vi "Slam.vi"() -> ()   [LabVIEW 2017]
uses:
  Control Globals.vi
  gyro/Gyro Globals.vi
  <vilib>/Platform/TimedLoop/XDataNode/wakeup.ctl
  <vilib>/Platform/TimedLoop/XDataNode/XDNodeRunTimeDep.lvlib
  <vilib>/Platform/TimedLoop/XDataNode/nitl_modes.ctl
  <vilib>/Platform/TimedLoop/XDataNode/timing_clust.ctl
  <vilib>/Platform/TimedLoop/XDataNode/XDataNode.xnode
  <vilib>/robotics/Steering/Steering Frame/NI_Robotics_Steering Frame.lvclass
  <vilib>/robotics/Steering/Steering Frame/Apply Steering Frame Velocity to Motors.vi
panel:
  out "Estimated Pose (Degrees)":cluster{"X":dbl, "Y":dbl, "R":dbl}
  in  "Desired Velocity":dbl[](array[numeric])=[0.0, 0.0, 0.0]
  out "Gyro Bias":cluster{"X":dbl, "Y":dbl, "Z":dbl}={"X"=0.039458598891488325, "Y"=-0.012762257416847495, "Z"=-0.06349169800034307}
  out "Slam Run Time":u32
  out "Intensity Graph":u16[][](graph)
  in  "stop":bool
  out "XY Graph":cluster{"X":dbl[], "Y":dbl[]}[](graph)
  out "Lidar Run Time":u32
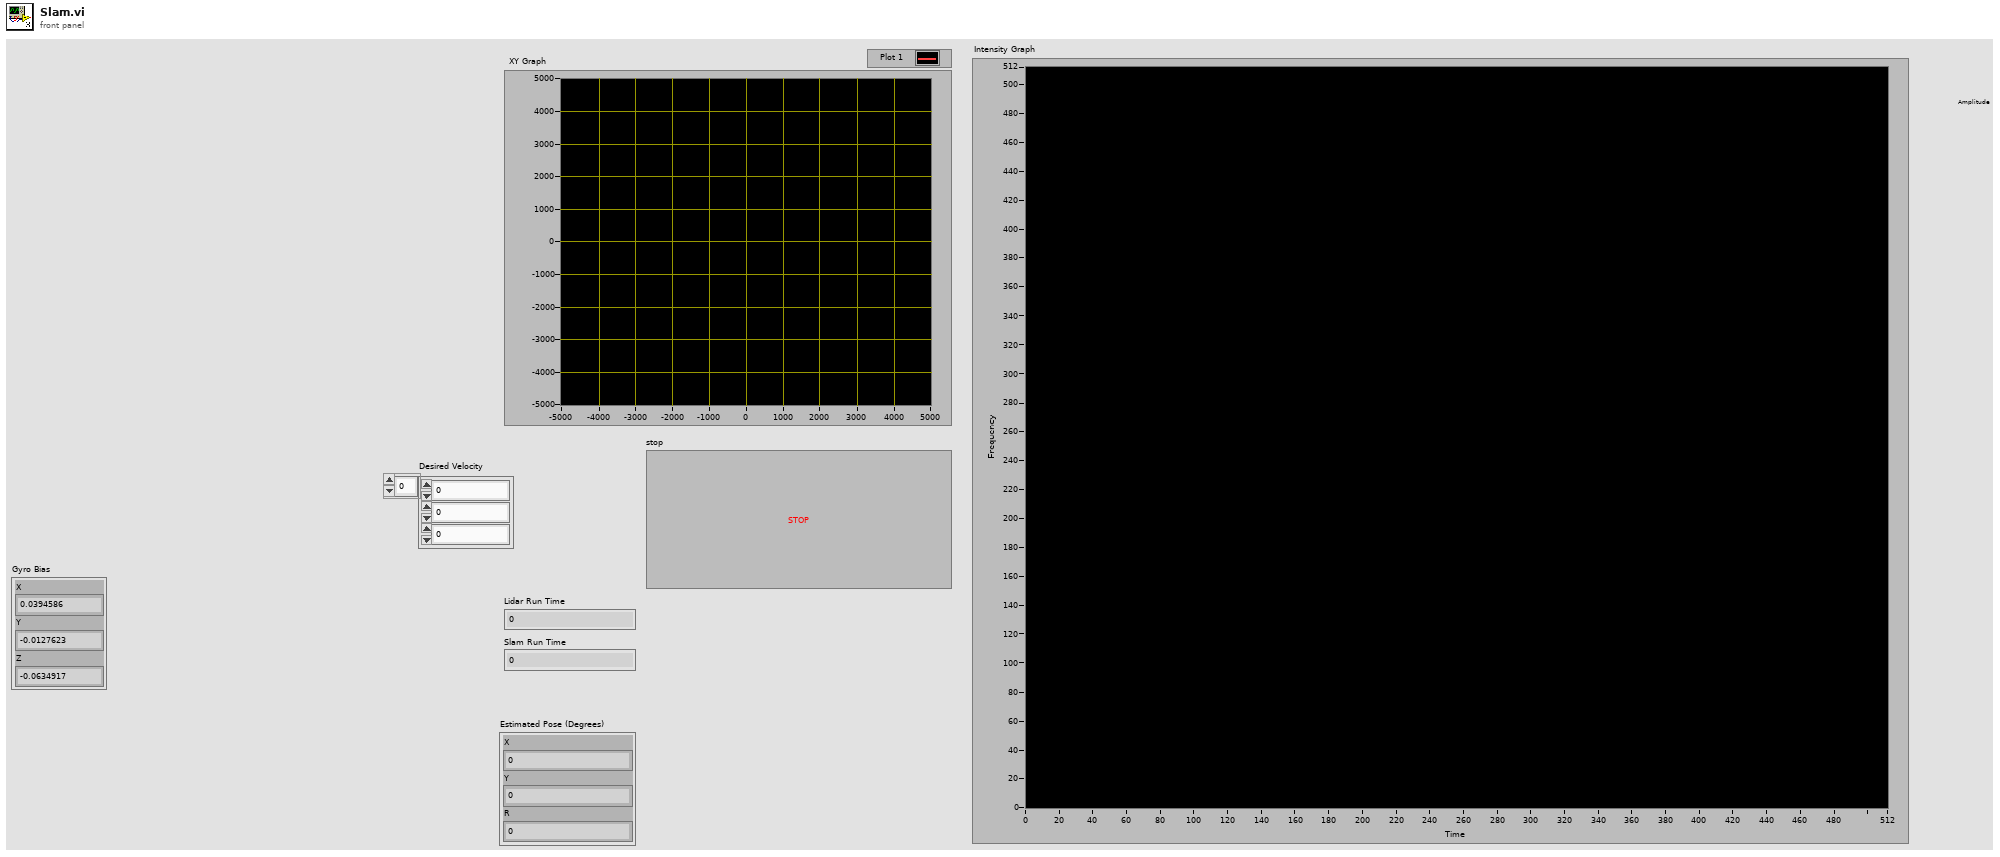
[diagram p1: front panel]
types:
  T1 = cluster{dbl[], dbl[], "Estimated Pose Delta":cluster{"X":dbl, "Y":dbl, "R":dbl}}
  T2 = typedef "XDNodeRunTimeDep.lvlib/timing_clust.ctl" = cluster{"Expected End [f-1]":u64, "Actual End [f-1]":u64, "Finished Late? [f-1]":bool, "Expected End [i-1]":u64, "Actual End [i-1]":u64, "Finished Late? [i-1]":bool, "Expected Start [i]":u64, "Actual Start [i]":u64, "Expected Start [f]":u64, "Actual Start [f]":u64, "Source Name":string, "Structure Name":string, "Period":i64, "Deadline":i64, "Offset":i64, "Start":i64, "Priority":i32, "Timeout":i32, "Mode":T3, "Wakeup Reason":T4, "Error":errorcluster, "Source Type":string, "Secondary Source Type":string, "Global End Time":u64, "Global Start Time":u64, "Frame Duration":u64, "Iteration Duration":u64, "Assigned CPU":i32, "I/O Scan Engine Mode":u32}
  T3 = typedef "XDNodeRunTimeDep.lvlib/nitl_modes.ctl" = enum32{"No Change", "Process missed periods, maintain original phase", "Discard missed periods, maintain original phase", "Process missed periods, ignore original phase", "Discard missed periods, ignore original phase"}
  T4 = typedef "XDNodeRunTimeDep.lvlib/wakeup.ctl" = enum32{"Normal", "Aborted", "Asynchronous wakeup", "Timing source error", "Timed loop error", "Timeout"}
  T5 = typedef "I2C.lvlib/I2C Reference.ctl" = cluster{"myRIO Reference":T6, "I2C Channels Enum":T10, "I2C Configuration":T11}
  T6 = typedef "myRIO Generic Hardware Reference.ctl" = cluster{"myRIO Model":T7, "myRIO Hardware Reference":T8}
  T7 = typedef "Hardware Version Enum.ctl" = enum16{"Unknown", "myRIO-1900", "myRIO-1950", "roboRIO", "NI ELVIS RIO CM"}
  T8 = typedef "myRIO v1.0 Reference.ctl" = cluster{"Generic FPGA Reference":T9, "Allow multiple opens":bool}
  T9 = typedef "Generic FPGA Reference.ctl" = refnum<k20>
  T10 = typedef "I2C Channels Enum.ctl" = enum16{"Not Connected", "A/I2C", "B/I2C", "I2C/I2C"}
  T11 = typedef "I2C.lvlib/I2C Configuration.ctl" = cluster{"I2C Transfer Rate":T12}
  T12 = typedef "I2C.lvlib/I2C Transfer Rate.ctl" = enum16{"Standard mode (100 kbps)", "Fast mode (400 kbps)"}
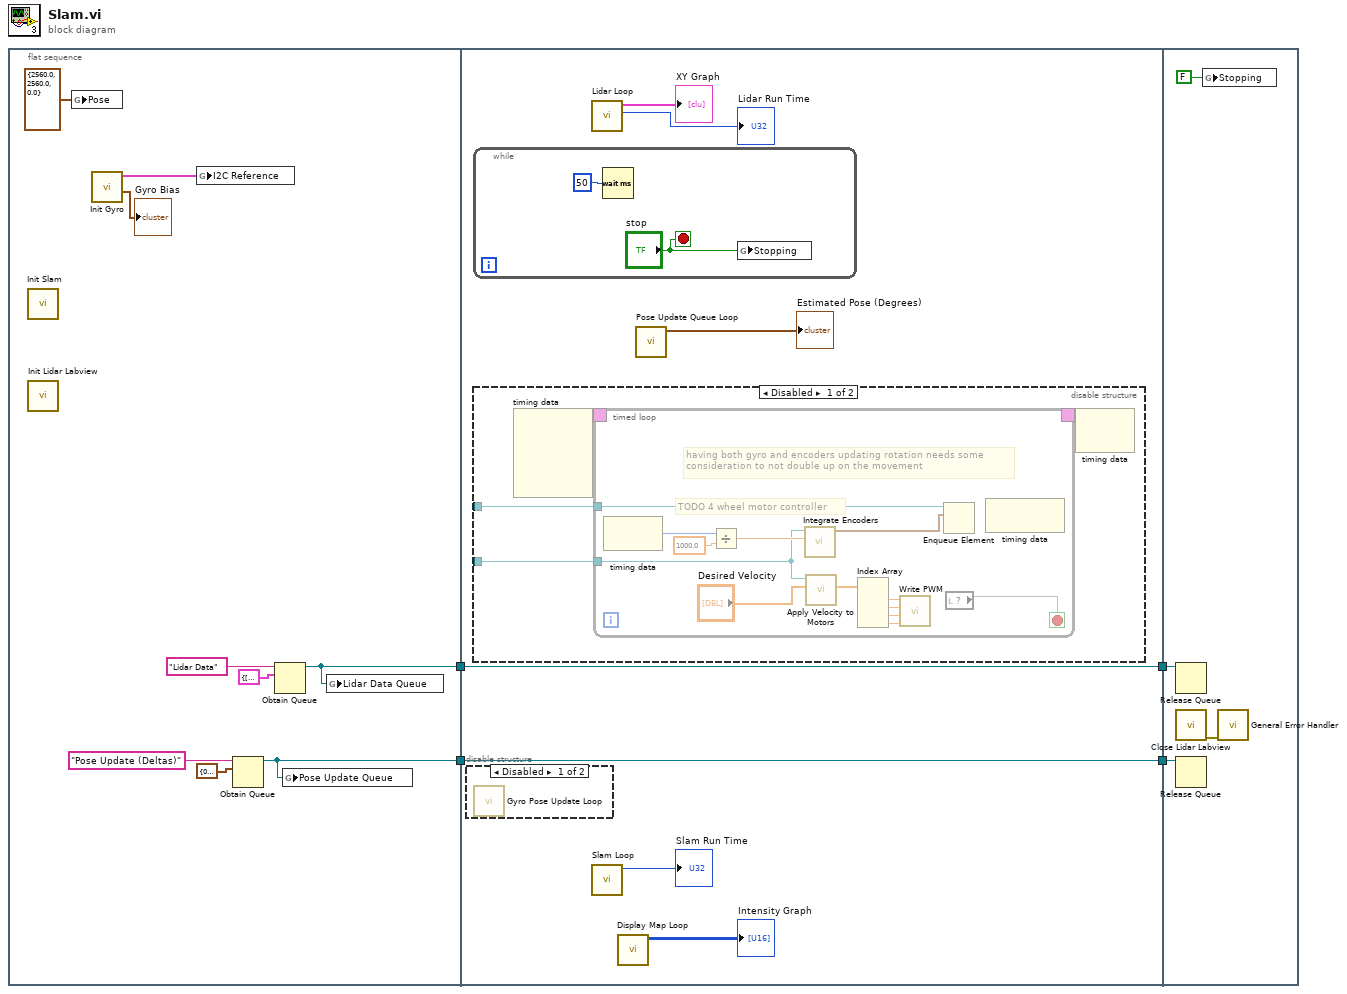
[diagram p0: block diagram]
diagram:
  n1 = flat-sequence {
    tunnel: [w8] -> w4
    tunnel: [w7] -> w3
    tunnel: w4 -> [w20]
    tunnel: w3 -> [w19]
    tunnel: [w20] -> w2
    tunnel: [w19] -> w1
    tunnel: w2 -> [w47]
    tunnel: w1 -> [w46]
    frame #0 {
      n2 = call "Init Slam.vi"() -> ()  [unwired: 12 in]
      n3 = call "Init Lidar Labview.vi"() -> ()  [unwired: 11 in, 1 out]
      n4 = global write "Control Globals.vi" "Pose"(cluster{"X":dbl, "Y":dbl, "R":dbl} {"X"=2560.0, "Y"=2560.0, "R"=0.0} ("Estimated Pose")) -> ()
      n5 = call "Init Gyro.vi"() -> ("Gyro Bias"=→"Gyro Bias":cluster{"X":dbl, "Y":dbl, "Z":dbl}, "I2C Ref Out"=w6:T5)  [unwired: 9 in, 1 out]
      n6 = global write "Gyro Globals.vi" "I2C Reference"(w6) -> ()
      n7 = Obtain Queue(name (unnamed)="Pose Update (Deltas)", element data type=cluster{"X":dbl, "Y":dbl, "R":dbl} {"X"=0.0, "Y"=0.0, "R"=0.0} ("Estimated Pose Delta")) -> (queue out=w7:refnum<queue>)  [unwired: 3 in, 2 out]
      n8 = Obtain Queue(name (unnamed)="Lidar Data", element data type=T1 {[], [], "Estimated Pose Delta"={"X"=0.0, "Y"=0.0, "R"=0.0}} ("output cluster")) -> (queue out=w8:refnum<queue>)  [unwired: 3 in, 2 out]
      n9 = global write "Control Globals.vi" "Pose Update Queue"(w7) -> ()
      n10 = global write "Control Globals.vi" "Lidar Data Queue"(w8) -> ()
    }
    frame #1 {
      n11 = disable-structure shown="Disabled" {
        frame Disabled {
          n12 = call "Gyro Pose Update Loop.vi"() -> ()  [unwired: 12 in]
        }
        frame Enabled {
        }
      }
      n13 = while {
        stop <- "stop" stop-if-true
        n14 = Wait (ms)(milliseconds to wait=u32 50) -> ()  [unwired: 1 out]
        n15 = global write "Control Globals.vi" "Stopping"("stop") -> ()
      }
      n16 = disable-structure shown="Disabled" {
        disable-tunnel: _ -> [w24 _]
        disable-tunnel: _ -> [w23 _]
        frame Disabled {
          n17 = node-c288() -> (w26:T2)  [unwired: 4 in]
          n18 = timed-loop {
            timing: w26 -> [_]
            timing-out: [_] -> w25
            tunnel: w24 -> [w32]
            tunnel: w23 -> [w28]
            stop <- w39 stop-if-true
            # "having both gyro and encoders updating rotation needs some\nconsideration to not double up on the movement"
            # "TODO 4 wheel motor controller"
            n19 = node-c288() -> (w36:i64)  [unwired: 1 in]
            n20 = Divide(x=w36, y=1000.0) -> (x/y=w37:dbl)
            n21 = call "Integrate Encoders.vi"("dt"=w37, "NI_Robotics_Steering Frame in"=w32) -> ("Estimated Pose Delta"=w27:cluster{dbl, dbl, dbl})  [unwired: 9 in]
            n22 = call-poly <vilib>:"Apply Velocity to Motors.vi"("steering frame velocity"="Desired Velocity", "steering frame in"=w32) -> ("ccw motor velocity setpoints"=w34:dbl[])  [unwired: 5 in, 4 out]
            n23 = Index Array(array=w34) -> (element #1=w35:dbl, element #2=w31:dbl, element #3=w30:dbl, element #4=w29:dbl)  [unwired: 4 in]
            n24 = call "Write PWM.vi"("Back Right"=w29, "Front Right"=w30, "Back Left"=w31, "Front Left"=w35) -> ()  [unwired: 8 in]
            n25 = Enqueue Element(queue=w28, element=w27) -> ()  [unwired: 2 in, 3 out]
            n26 = local read item#-1() -> (w39)
            n27 = node-c288() -> ()  [unwired: 1 in, 1 out]
          }
          n28 = node-c288(w25) -> ()  [unwired: 1 out]
        }
        frame Enabled {
        }
      }
      n29 = call "Lidar Loop.vi"() -> ("Lidar Run Time"=→"Lidar Run Time":u32, "XY Graph"=→"XY Graph":cluster{"X":dbl[], "Y":dbl[]}[])  [unwired: 10 in]
      n30 = call "Slam Loop.vi"() -> ("slam run time"=→"Slam Run Time":u32)  [unwired: 11 in]
      n31 = call "Display Map Loop.vi"() -> ("Intensity Graph"=→"Intensity Graph":u16[][])  [unwired: 11 in]
      n32 = call "Pose Update Queue Loop.vi"() -> ("Estimated Pose (Degrees)"=→"Estimated Pose (Degrees)":cluster{"X":dbl, "Y":dbl, "R":dbl})  [unwired: 11 in]
    }
    frame #2 {
      n33 = Release Queue(queue=w47) -> ()  [unwired: 2 in, 3 out]
      n34 = call "Close Lidar Labview.vi"() -> ("error out"=w48:errorcluster)  [unwired: 11 in]
      n35 = Release Queue(queue=w46) -> ()  [unwired: 2 in, 3 out]
      n36 = global write "Control Globals.vi" "Stopping"(FALSE) -> ()
      n37 = call <vilib>:"General Error Handler.vi"("error in (no error)"=w48) -> ()  [unwired: 10 in, 5 out]
    }
  }
